vi "CtoF.vi"(0 "Celsius":u8(slide) scale=0.0..100.0) -> (7 "Fahrenheit":dbl(slide) scale=0.0..100.0)   [LabVIEW 2022 SP3]
panel:
  out "Numeric 2":dbl
  out "Numeric":dbl
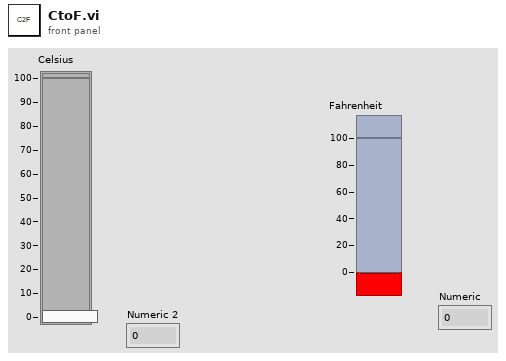
[diagram p1: front panel]
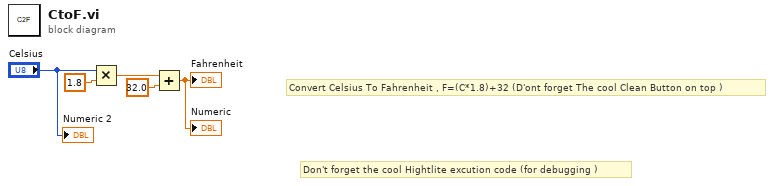
[diagram p0: block diagram]
diagram:
  # "Don't forget the cool Hightlite excution code (for debugging )"
  # "Convert Celsius To Fahrenheit , F=(C*1.8)+32 (D'ont forget The cool Clean Button on top )"
  n1 = Multiply(x="Celsius", y=1.8) -> (x*y=w3:dbl)
  n2 = Add(x=w3, y=32.0) -> (x+y=→"Fahrenheit" →"Numeric":dbl)
  "Numeric 2" <- "Celsius"
